vi "Vision.vi"() -> (2 "Center":cluster{dbl, dbl}, 3 "seen":bool=TRUE)   [LabVIEW 2016]
uses:
  Robot Global Data.vi
panel:
  out "Rectangle":T1
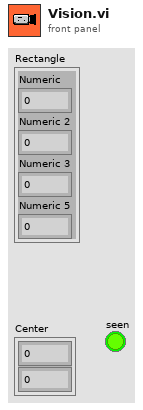
[diagram p1: front panel]
types:
  T1 = cluster{"Numeric":dbl, "Numeric 2":dbl, "Numeric 3":dbl, "Numeric 5":dbl}
  T2 = cluster{"Distance (ft)":dbl, "Score":dbl, "Normalized":cluster{"Center":cluster{dbl, dbl}, "Rectangle":cluster{"Numeric":dbl, "Numeric 2":dbl, "Numeric 3":dbl, "Numeric 5":dbl}}, "Pixels":cluster{"Center":cluster{dbl, dbl}, "Rectangle":cluster{"Numeric":dbl, "Numeric 2":dbl, "Numeric 3":dbl, "Numeric 5":dbl}}}
  T3 = cluster{"Center":cluster{dbl, dbl}, "Rectangle":cluster{"Numeric":dbl, "Numeric 2":dbl, "Numeric 3":dbl, "Numeric 5":dbl}}
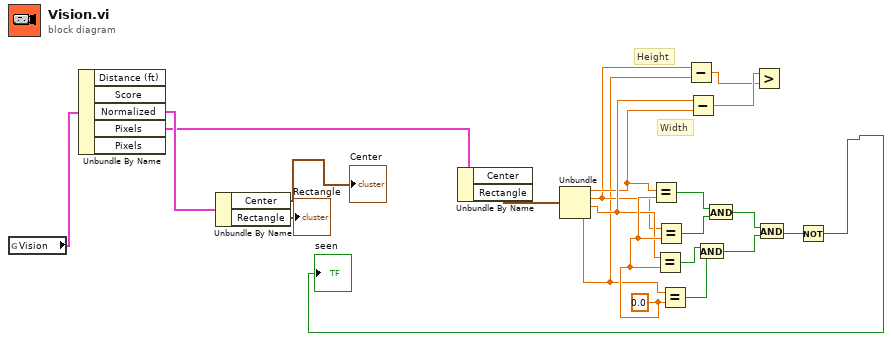
[diagram p0: block diagram]
diagram:
  w9 = 0.0 ("y")
  # "Width"
  # "Height"
  n1 = global read "Robot Global Data.vi" "Vision"() -> (w20:T2)
  n2 = Unbundle By Name(w20) -> ("Normalized"=w21:T3, "Pixels"=w18:T3)  [unwired: 3 out]
  n3 = Unbundle By Name(w21) -> ("Center"=→"Center":cluster{dbl, dbl}, "Rectangle"=→"Rectangle":T1)
  n4 = Unbundle By Name(w18) -> ("Rectangle"=w17:T1)  [unwired: 1 out]
  n5 = Unbundle(w17) -> ("Numeric"=w6:dbl, "Numeric 2"=w5:dbl, "Numeric 3"=w7:dbl, "Numeric 5"=w4:dbl)
  n6 = Equal?(x=w6, y=w9) -> (x = y?=w14:bool)
  n7 = Equal?(x=w7, y=w9) -> (x = y?=w12:bool)
  n8 = Equal?(x=w5, y=w9) -> (x = y?=w13:bool)
  n9 = Equal?(x=w4, y=w9) -> (x = y?=w11:bool)
  n10 = Subtract(x=w5, y=w4) -> (x-y=w2:dbl)
  n11 = Subtract(x=w7, y=w6) -> (x-y=w3:dbl)
  n12 = And(x=w12, y=w11) -> (x .and. y?=w16:bool)
  n13 = And(x=w14, y=w13) -> (x .and. y?=w15:bool)
  n14 = Greater?(x=w3, y=w2) -> ()  [unwired: 1 out]
  n15 = And(x=w15, y=w16) -> (x .and. y?=w10:bool)
  n16 = Not(x=w10) -> (.not. x?=→"seen":bool)
